vi "Read Construct String Camera Status.lvclass.vi"(8 "error in (no error)":errorcluster, 11 "RxTxCamera in":refnum<class "RxTxCamera.lvclass">) -> (0 "error out":errorcluster, 2 "Construct String Camera Status.lvclass":refnum<class "Construct String Camera Status.lvclass">, 3 "RxTxCamera out":refnum<class "RxTxCamera.lvclass">)   [LabVIEW 2018, in "RxTxCamera.lvclass"]
doc: "Este VI faz a leitura da classe construtora do status da câmera."
uses:
  RxTxCamera.lvclass
  Construct String Camera Status/Construct String Camera Status.lvclass
  RxTxCamera.lvclass/RxTxCamera.ctl
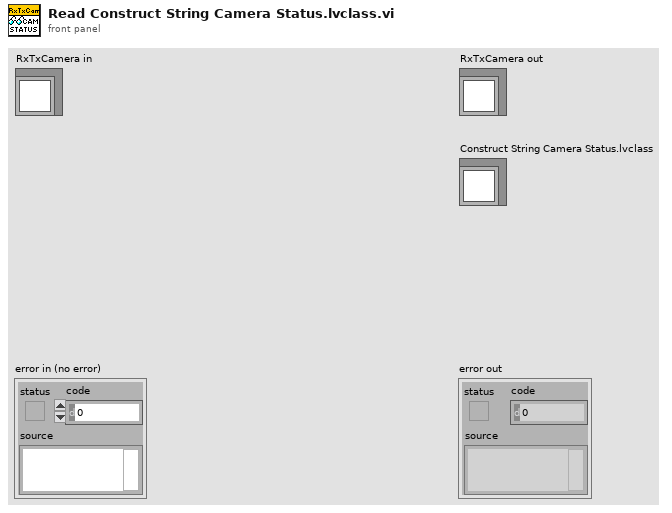
[diagram p1: front panel]
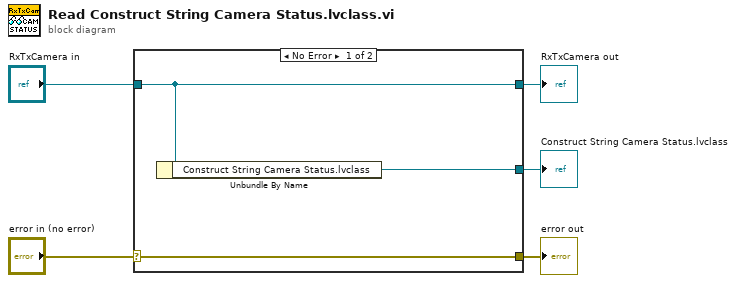
[diagram p0: block diagram]
diagram:
  n1 = case shown="No Error" "error in (no error)" {
    selector: "error in (no error)" -> [w8 w9]
    tunnel: [w8 w9] -> w4
    tunnel: [w7 w10] -> w2
    tunnel: "RxTxCamera in" -> [w7 w10]
    tunnel: [w6 _] -> w1
    frame No Error {
      n2 = Unbundle By Name(w7) -> ("Construct String Camera Status.lvclass"=w6:refnum<class "Construct String Camera Status.lvclass">)
    }
    frame Error {
    }
  }
  "error out" <- w4
  "RxTxCamera out" <- w2
  "Construct String Camera Status.lvclass" <- w1
